vi "UpdateImage.vi"(0 "Show Image":bool, 1 "Retrace":bool, 2 "Update Data":T1) -> ()   [LabVIEW 2009]
panel:
  out "error out":errorcluster
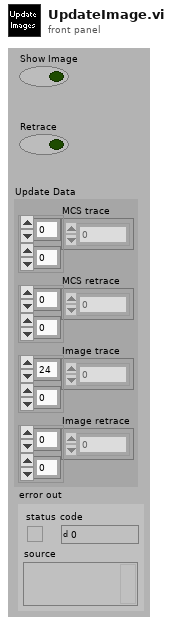
[diagram p1: front panel]
types:
  T1 = cluster{"MCS trace":u32[][], "MCS retrace":u32[][], "Image trace":u32[][], "Image retrace":u32[][]}
  T2 = typedef "DAQLinescanVisualization.ctt" = cluster{"Threshold":u32, "Trace Window #":u32, "IMAQ Trace":T3, "Retrace Window #":u32, "IMAQ Retrace":T3}
  T3 = typedef "IMAQ Image.ctl" = refnum<image>
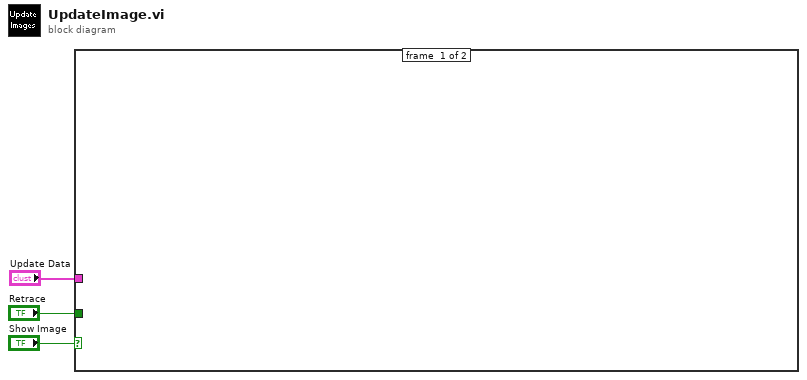
[diagram p0: block diagram]
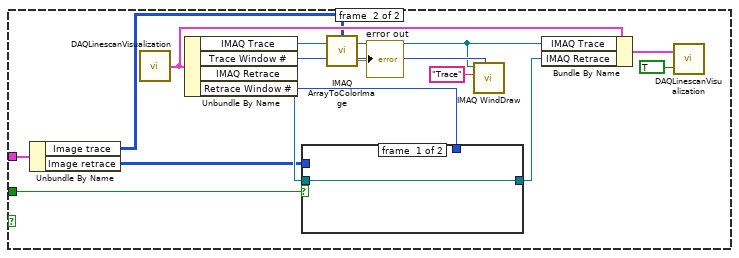
[diagram p2: hidden frame]
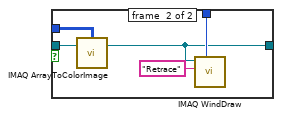
[diagram p3: hidden frame]
diagram:
  n1 = case shown="True" "Show Image" {
    tunnel: "Retrace" -> [_ w14]
    tunnel: "Update Data" -> [_ w10]
    frame #0 {
    }
    frame #1 {
      n2 = Unbundle By Name(w10) -> ("Image trace"=w5:u32[][], "Image retrace"=w11:u32[][])
      n3 = call "DAQLinescanVisualization.vi"() -> ("Visualization (output)"=w17:T2)  [unwired: 2 in]
      n4 = Unbundle By Name(w17) -> ("IMAQ Trace"=w18:T3, "Trace Window #"=w8:u32, "IMAQ Retrace"=w13:T3, "Retrace Window #"=w9:u32)
      n5 = case shown="True" w14 {
        tunnel: w13 -> [w19 w24]
        tunnel: [w19 w21] -> w12
        tunnel: w11 -> [_ w23]
        tunnel: w9 -> [_ w22]
        frame #0 {
        }
        frame #1 {
          n6 = call "IMAQ ArrayToColorImage"("Image Pixels (U32)"=w23, "Image"=w24) -> ("Image Out"=w21:T3)  [unwired: 3 in, 1 out]
          n7 = call "IMAQ WindDraw"("Window Number (0...15)"=w22, "Title"="Retrace", "Image"=w21) -> ()  [unwired: 7 in, 2 out]
        }
      }
      n8 = call "IMAQ ArrayToColorImage"("Image Pixels (U32)"=w5, "Image"=w18) -> ("Image Out"=w7:T3, "error out"=→"error out":errorcluster)  [unwired: 3 in]
      n9 = call "IMAQ WindDraw"("Window Number (0...15)"=w8, "Title"="Trace", "Image"=w7) -> ()  [unwired: 7 in, 2 out]
      n10 = Bundle By Name(cluster=w17, "IMAQ Trace"=w7, "IMAQ Retrace"=w12) -> (w16:T2)
      n11 = call "DAQLinescanVisualization.vi"("Get/Set"=TRUE, "Visualization (input)"=w16) -> ()  [unwired: 1 out]
    }
  }
